vi "ROS_Master_checkNode.vi"(2 "PubSub":T2, 3 "ROS_Master in":T1) -> (1 "ROS_Master out":T1)   [LabVIEW 2015]
uses:
  ROS_Topic.ctl
  ROS_Master.ctl
  ROS_Node.ctl
  ROS_Service.ctl
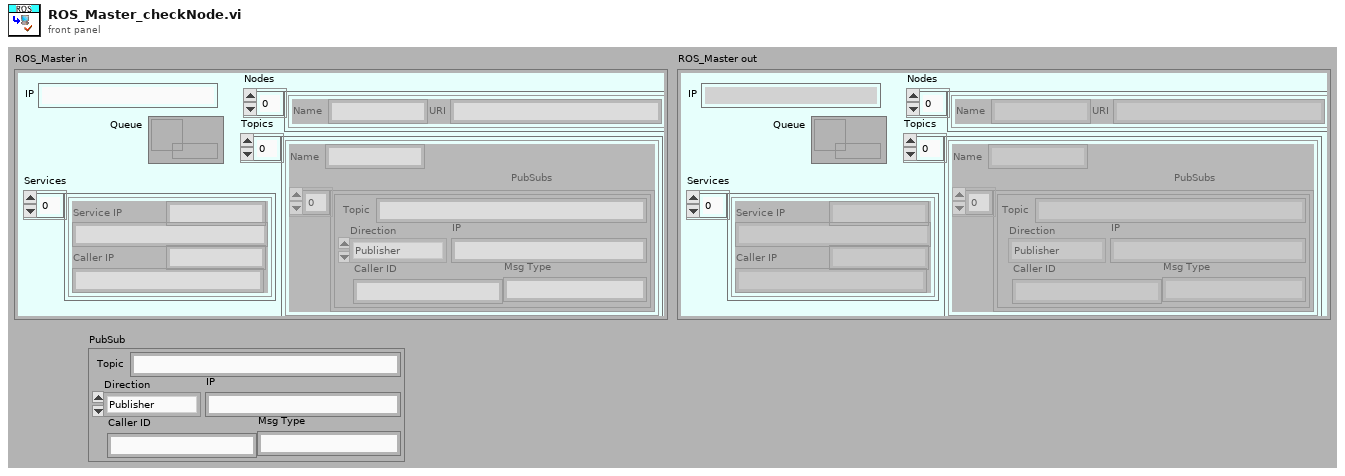
[diagram p1: front panel]
types:
  T1 = typedef "ROS_Master.ctl" = cluster{"IP":string, "Topics":cluster{"Name":string, "PubSubs":T2[]}[], "Nodes":T3[], "Services":T4[], "Queue":refnum<queue>}
  T2 = typedef "ROS_Topic.ctl" = cluster{"Caller ID":string, "IP":string, "Msg Type":string, "Direction":enum16{"Publisher", "Subscriber"}, "Topic":string}
  T3 = typedef "ROS_Node.ctl" = cluster{"Name":string, "URI":string}
  T4 = typedef "ROS_Service.ctl" = cluster{"Service":string, "Service IP":string, "Caller IP":string, "Caller ID":string}
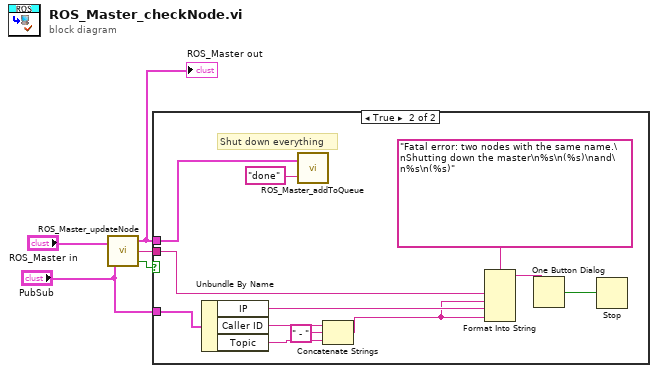
[diagram p0: block diagram]
diagram:
  n1 = call "ROS_Master_updateNode.vi"("ROS_Master in"="ROS_Master in", "PubSub"="PubSub") -> ("ROS_Master out"=w2:T1, "Shutdown URI"=w5:string, "shutdown needed?"=w4:bool)
  "ROS_Master out" <- w2
  n2 = case shown="True" w4 {
    tunnel: w5 -> [_ w12]
    tunnel: w2 -> [_ w8]
    tunnel: "PubSub" -> [_ w14]
    frame False {
    }
    frame True {
      # "Shut down everything"
      n3 = Unbundle By Name(w14) -> ("IP"=w13:string, "Caller ID"=w10:string, "Topic"=w11:string)
      n4 = call "ROS_Master_addToQueue.vi"("Message"="done" ("format string"), "ROS_Master in"=w8) -> ()  [unwired: 2 in]
      n5 = Concatenate Strings(w10, " - " ("string"), w11) -> (w7:string)
      n6 = Format Into String(format string="Fatal error: two nodes with the same name.\nShutting down the master\n%s\n(%s)\nand\n%s\n(%s)" ("message"), w12, w7, w13, w7) -> (resulting string=w15:string)  [unwired: 2 in, 1 out]
      n7 = One Button Dialog(message=w15) -> (true=w6:bool)  [unwired: 1 in]
      n8 = Stop(stop? (T)=w6) -> ()
    }
  }
